vi "更新软件.vi"(8 "error in (no error)":errorcluster, 11 "远端地址":string="/updatefiles/OneStation/V4/一体化微型水质监测站.zip") -> (0 "error out":errorcluster)   [LabVIEW 2016, in "数据传输系统-03.lvlib" / "update.lvlib" / "http client.lvclass"]
uses:
  http client.lvclass
  update.lvlib
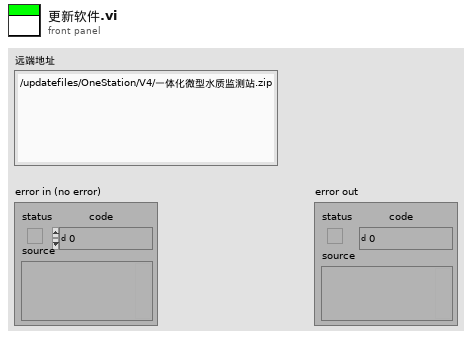
[diagram p1: front panel]
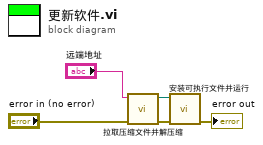
[diagram p0: block diagram]
diagram:
  n1 = call "拉取压缩文件并解压缩.vi"("error in (no error)"="error in (no error)", "远端地址"="远端地址") -> ("error out"=w4:errorcluster, "文件路径"=w5:path)  [unwired: 8 in]
  n2 = call "安装可执行文件并运行.vi"("error in (no error)"=w4, "源路径"=w5) -> ("error out"=→"error out":errorcluster)  [unwired: 9 in]
